vi "Data1.set.vi"(8 "error in (no error)":errorcluster, 10 "Data1":u8, 11 "midi-file-event.midi in":refnum<class "midi-file-event.midi.lvclass">) -> (0 "error out":errorcluster, 3 "midi-file-event.midi out":refnum<class "midi-file-event.midi.lvclass">)   [LabVIEW 2020, in "midi-file-event.midi.lvclass"]
uses:
  midi-file-event.midi.lvclass
  midi-file-event.midi.lvclass/midi-file-event.midi.ctl
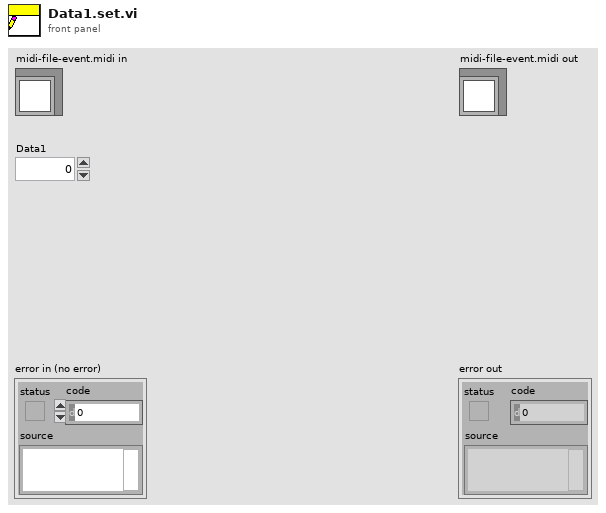
[diagram p1: front panel]
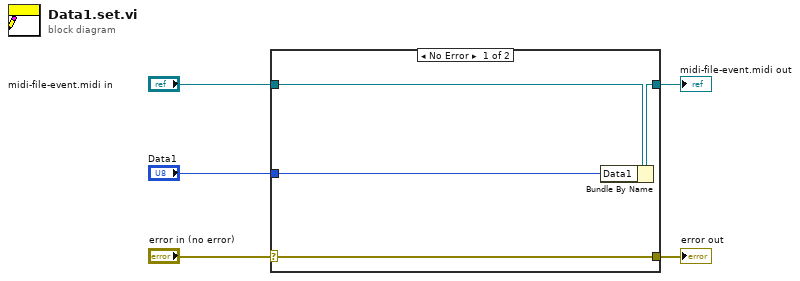
[diagram p0: block diagram]
diagram:
  n1 = case shown="No Error" "error in (no error)" {
    selector: "error in (no error)" -> [w9 w10]
    tunnel: [w9 w10] -> w4
    tunnel: [w7 w11] -> w2
    tunnel: "midi-file-event.midi in" -> [w8 w11]
    tunnel: "Data1" -> [w6 _]
    frame No Error {
      n2 = Bundle By Name(cluster=w8, "Data1"=w6) -> (w7:refnum<class "midi-file-event.midi.lvclass">)
    }
    frame Error {
    }
  }
  "error out" <- w4
  "midi-file-event.midi out" <- w2
